vi "GetACPadErrors.vi"() -> ()   [LabVIEW 2018]
uses:
  <vilib>/userdefined/High Color/IMAQdx.ctl
  <vilib>/Utility/file.llb/Read Delimited Spreadsheet (DBL).vi
  <vilib>/Utility/file.llb/Read Delimited Spreadsheet (I64).vi
  <vilib>/Utility/file.llb/Write Delimited Spreadsheet (DBL).vi
  <vilib>/vision/driver/NI_Vision_Acquisition_Software.lvlib
  <vilib>/vision/NI_Vision_Development_Module.lvlib
panel:
  in  "Sensor":string(combo)="R0Hamamatsu"
  in  "Begin":bool
  out "Image Out":T1(plugin-control)
  out "Pattern Matched Image":T1(plugin-control)
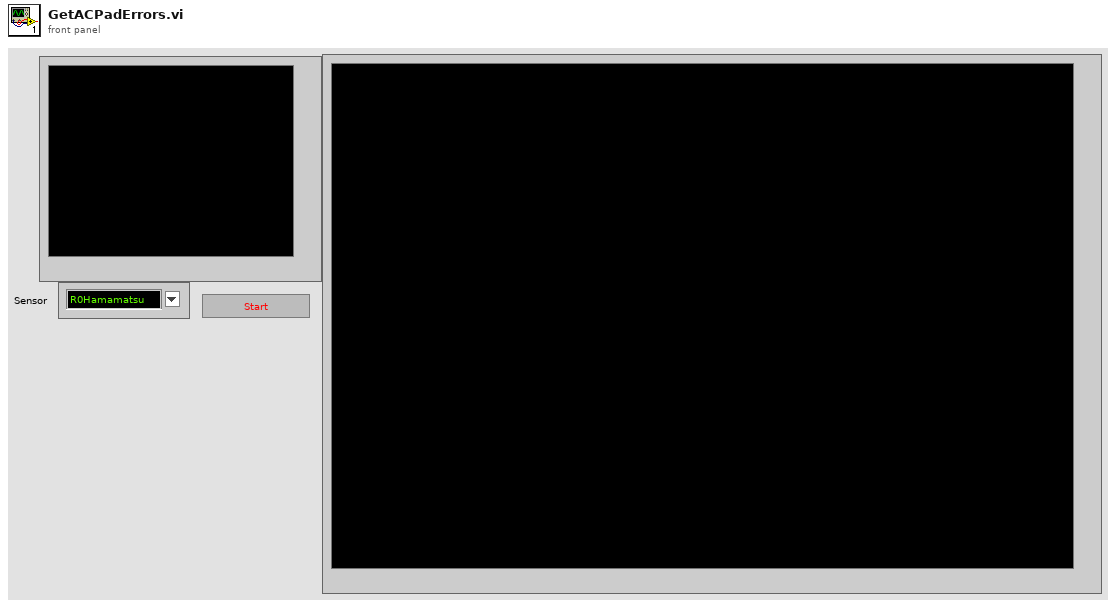
[diagram p1: front panel]
types:
  T1 = typedef "IMAQ Image.ctl" = refnum<image>
  T2 = typedef "Image Type" = u32
  T3 = typedef "IMAQdx.ctl" = refnum<k21>
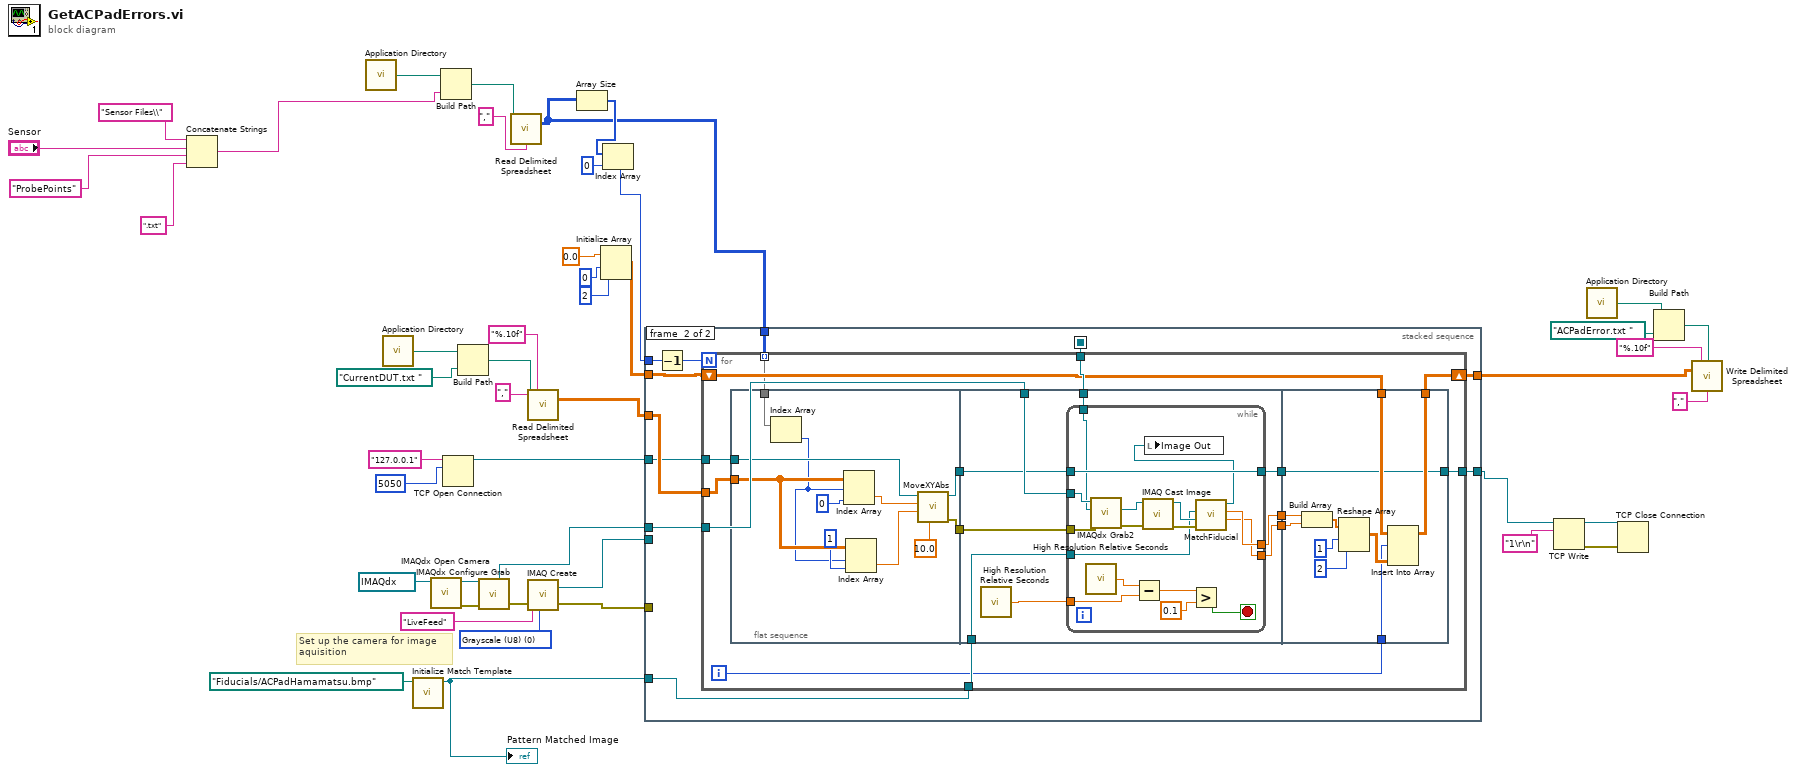
[diagram p0: block diagram]
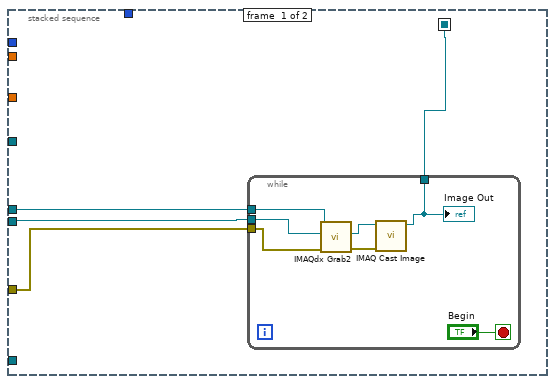
[diagram p2: hidden frame]
diagram:
  w36 = T2 0 items=["Grayscale (U8)", "Grayscale (I16)", "Grayscale (SGL)", "Complex (CSG)", "RGB (U32)", "HSL (U32)", "RGB (U64)", "Grayscale (U16)"] ("Image Type")
  # "Set up the camera for image \naquisition"
  n1 = Concatenate Strings("Sensor Files\\" ("string"), "Sensor", "ProbePoints" ("string"), ".txt" ("string")) -> (w3:string)
  n2 = call <vilib>:"Application Directory.vi"() -> ("Application Directory"=w10:path)
  n3 = call <vilib>:"Application Directory.vi"() -> ("Application Directory"=w43:path)
  n4 = call "Initialize Match Template.vi"("base path"=path "Fiducials/ACPadHamamatsu.bmp") -> ("Pattern Matched Image"=w35:T1)  [unwired: 10 in]
  "Pattern Matched Image" <- w35
  n5 = call <vilib>:"IMAQdx Open Camera.vi"("Session In"=T3 "cam0") -> ("error out"=w39:errorcluster, "Session Out"=w40:T3)  [unwired: 9 in]
  n6 = Build Path(base path=w10, name or relative path=w3) -> (appended path=w11:path)
  n7 = TCP Open Connection(address="127.0.0.1", remote port or service name=u16 5050) -> (connection ID=w18:refnum<k5>)  [unwired: 3 in, 1 out]
  n8 = Build Path(base path=w43, name or relative path=path "CurrentDUT.txt " ("file path (dialog if empty)")) -> (appended path=w44:path)
  n9 = call <vilib>:"IMAQdx Configure Grab.vi"("error in"=w39, "Session In"=w40) -> ("error out"=w37:errorcluster, "Session Out"=w34:T3)  [unwired: 8 in]
  n10 = call-poly <vilib>:"Read Delimited Spreadsheet.vi"("file path (dialog if empty)"=w11, "delimiter (\\t)"="," ("delimiter (\\t)")) -> ("all rows"=w6:i64[][])  [unwired: 8 in, 5 out]
  n11 = call-poly <vilib>:"Read Delimited Spreadsheet.vi"("file path (dialog if empty)"=w44, "format (%.3f)"="%.10f", "delimiter (\\t)"="," ("delimiter (\\t)")) -> ("all rows"=w13:dbl[][])  [unwired: 7 in, 5 out]
  n12 = call "IMAQ Create"("Image Name"="LiveFeed", "Image Type"=w36, "error in (no error)"=w37) -> ("New Image"=w33:T1, "error out"=w32:errorcluster)  [unwired: 2 in]
  n13 = Array Size(array=w6) -> (size(s)=w9:i32[])
  n14 = Initialize Array(0.0 ("element"), 0 ("dimension size"), 2 ("dimension size")) -> (w22:dbl[][])
  n15 = Index Array(array=w9, index=0) -> (element=w7:i32)
  n16 = stacked-sequence {
    seq-local: [w47 _] -> [_ w67]
    tunnel: w35 -> [_ w68]
    tunnel: w34 -> [w50 w66]
    tunnel: w33 -> [w49 _]
    tunnel: w32 -> [w48 _]
    tunnel: w13 -> [_ w63]
    tunnel: [_ w65] -> w23
    tunnel: w22 -> [_ w64]
    tunnel: w18 -> [_ w62]
    tunnel: [_ w61] -> w14
    tunnel: w7 -> [_ w60]
    tunnel: w6 -> [_ w58]
    frame #0 {
      n17 = while {
        tunnel: w50 -> [w56]
        tunnel: w48 -> [w55]
        tunnel: w49 -> [w54]
        tunnel: [w51] -> w47
        stop <- "Begin" stop-if-true
        n18 = call <vilib>:"IMAQdx Grab2.vi"("error in"=w55, "Image In"=w54, "Session In"=w56) -> ("error out"=w52:errorcluster, "Image Out"=w53:T1)  [unwired: 5 in, 2 out]
        n19 = call "IMAQ Cast Image"("error in (no error)"=w52, "Image Src"=w53) -> ("Image Dst Out"=w51:T1)  [unwired: 8 in, 1 out]
        "Image Out" <- w51
      }
    }
    frame #1 {
      n20 = Decrement(x=w60) -> (x-1=w59:i32)
      n21 = for {
        N: w59 -> [_]
        tunnel: w68 -> [w83]
        tunnel: w67 -> [w82]
        tunnel: w66 -> [w81]
        shift-right: [w78] -> w65
        shift-left: w64 -> [w77]
        tunnel: w63 -> [w76]
        tunnel: w62 -> [w74]
        tunnel: [w70] -> w61
        tunnel: w58 -> [w69] mode=indexing
        i -> [w75]
        n22 = flat-sequence {
          tunnel: w76 -> [w92]
          tunnel: w74 -> [w89]
          tunnel: [w87] -> w73
          tunnel: [w86] -> w72
          tunnel: w69 -> [w85]
          tunnel: w83 -> [w102]
          tunnel: w82 -> [w101]
          tunnel: w81 -> [w100]
          tunnel: [w98] -> w80
          tunnel: [w99] -> w79
          tunnel: w73 -> [w97]
          tunnel: w72 -> [w96]
          tunnel: [w95] -> w71
          tunnel: [w128] -> w78
          tunnel: w80 -> [w127]
          tunnel: w79 -> [w126]
          tunnel: w75 -> [w125]
          tunnel: w77 -> [w122]
          tunnel: [w121] -> w70
          tunnel: w71 -> [w121]
          frame #0 {
            n23 = Index Array(array=w85) -> (element=w84:i64)  [unwired: 1 in]
            n24 = Index Array(array=w92, index (row)=w84, index (col)=0 ("index")) -> (element=w94:dbl)
            n25 = Index Array(array=w92, index (row)=w84, index (col)=1 ("index")) -> (element=w93:dbl)
            n26 = call "MoveXYAbs.vi"("%Speed"=10.0, "Y"=w93, "X"=w94, "connection ID 2"=w89) -> ("error out"=w87:errorcluster, "connection ID"=w86:refnum<k5>)  [unwired: 6 in]
          }
          frame #1 {
            n27 = call <vilib>:"High Resolution Relative Seconds.vi"() -> ("relative seconds"=w103:dbl)
            n28 = while {
              tunnel: w103 -> [w117]
              tunnel: w102 -> [w106]
              tunnel: w97 -> [w111]
              tunnel: w101 -> [w110]
              tunnel: w100 -> [w120]
              tunnel: [w114] -> w98
              tunnel: [w113] -> w99
              tunnel: w96 -> [w112]
              tunnel: [w112] -> w95
              stop <- w119 stop-if-true
              n29 = call <vilib>:"High Resolution Relative Seconds.vi"() -> ("relative seconds"=w118:dbl)
              n30 = call <vilib>:"IMAQdx Grab2.vi"("error in"=w111, "Image In"=w110, "Session In"=w120) -> ("error out"=w109:errorcluster, "Image Out"=w104:T1)  [unwired: 5 in, 2 out]
              n31 = Subtract(x=w118, y=w117) -> (x-y=w116:dbl)
              n32 = call "IMAQ Cast Image"("error in (no error)"=w109, "Image Src"=w104) -> ("error out"=w108:errorcluster, "Image Dst Out"=w107:T1)  [unwired: 8 in]
              n33 = Greater?(x=w116, y=0.1) -> (0:w119:bool)
              n34 = call "MatchFiducial.vi"("error in"=w108, "Image In"=w107, "Template Image"=w106) -> ("Y (um)"=w113:dbl, "X (um)"=w114:dbl, "Image Out"=w105:T1)  [unwired: 3 in, 3 out]
              n35 = local write "Image Out"(w105) -> ()
            }
          }
          frame #2 {
            n36 = Build Array(w127, w126) -> (w130:dbl[])
            n37 = Reshape Array(w130, 1 ("dimension size"), 2 ("dimension size")) -> (w129:dbl[][])
            n38 = Insert Into Array(array=w122, index (row)=w125, new element=w129) -> (w128:dbl[][])  [unwired: 1 in]
          }
        }
      }
    }
  }
  n39 = TCP Write(connection ID=w14, data in="1\r\n") -> (connection ID out=w16:refnum<k5>, error out=w17:errorcluster)  [unwired: 2 in, 1 out]
  n40 = call <vilib>:"Application Directory.vi"() -> ("Application Directory"=w27:path)
  n41 = TCP Close Connection(connection ID=w16, error in (no error)=w17) -> ()  [unwired: 1 in, 2 out]
  n42 = Build Path(base path=w27, name or relative path=path "ACPadError.txt " ("file path (dialog if empty)")) -> (appended path=w26:path)
  n43 = call-poly <vilib>:"Write Delimited Spreadsheet.vi"("file path (dialog if empty)"=w26, "format (%.3f)"="%.10f", "2D data"=w23, "delimiter (\\t)"="," ("delimiter (\\t)")) -> ()  [unwired: 10 in, 2 out]
